vi "Build Command Frame.vi"(0 "RFFE Standard Command in":refnum<class "RFFE Standard Command.lvclass">, 11 "error in (no error)":errorcluster) -> (4 "RFFE Standard Command out":refnum<class "RFFE Standard Command.lvclass">, 6 "Command Frame":u8[](array[numeric]), 15 "error out":errorcluster)   [LabVIEW 2018, in "MIPI RFFE API.lvlib" / "RFFE Standard Command.lvclass"]
uses:
  RFFE Standard Command.lvclass
  C:/Users/semoore/Projects/mipi-rffe-labview-oop/Command/RFFE Command.lvclass
  Command/RFFE Command.lvclass/RFFE Command.ctl
  Command/Get Slave Address.vi
  Command/Get Register Address.vi
  Command/Get Command Bits.vi
  MIPI RFFE API.lvlib
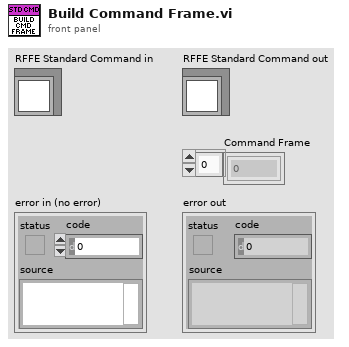
[diagram p1: front panel]
types:
  T1 = typedef "RFFE Commands.lvlib/Slave Address.ctl" = u8
  T2 = typedef "RFFE Commands.lvlib/Register Address.ctl" = u16
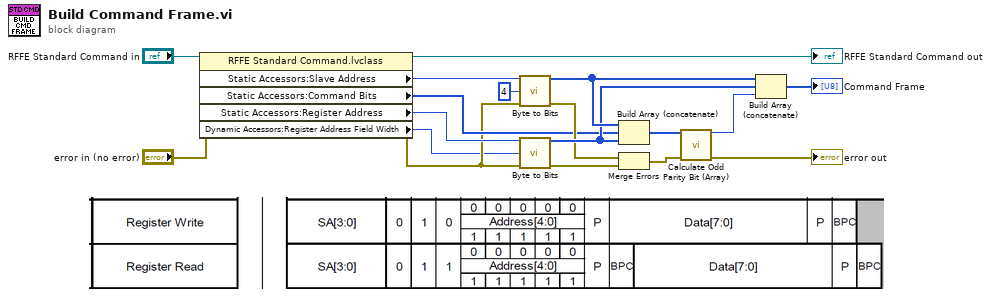
[diagram p0: block diagram]
diagram:
  n1 = property class="RFFE Standard Command.lvclass"(reference="RFFE Standard Command in", error in="error in (no error)") -> (reference out=→"RFFE Standard Command out":refnum<class "RFFE Standard Command.lvclass">, error out=w2:errorcluster, "Static Accessors:Slave Address"=w12:T1, "Static Accessors:Command Bits"=w3:u8[], "Static Accessors:Register Address"=w5:T2, "Dynamic Accessors:Register Address Field Width"=w1:i32)
  n2 = call "Byte to Bits.vi"("Byte"=w12, "Bit Width"=4, "error in (no error)"=w2) -> ("Bits"=w8:u8[], "error out"=w4:errorcluster)  [unwired: 11 in]
  n3 = call "Byte to Bits.vi"("Byte"=w5, "Bit Width"=w1, "error in (no error)"=w2) -> ("Bits"=w6:u8[], "error out"=w10:errorcluster)  [unwired: 11 in]
  n4 = Build Array (concatenate)(w8, w3, w6) -> (w11:u8[])
  n5 = Merge Errors(w4, w10) -> (w9:errorcluster)
  n6 = call "Calculate Odd Parity Bit (Array).vi"("Bytes"=w11, "error in (no error)"=w9) -> ("Odd Parity Bit"=w7:u8, "error out"=→"error out":errorcluster)  [unwired: 12 in]
  n7 = Build Array (concatenate)(w8, w6, w7) -> (→"Command Frame":u8[])
